vi "Email Alert (SubVI).vi"(6 "Password":string, 9 "Email":string, 10 "Phone Number":string, 11 "Carrier":enum16{"Sprint", "Verizon", "AT&T", "T-Mobile"}(ring)) -> (0 "error out":errorcluster)   [LabVIEW 2020]
uses:
  <vilib>/smtpClient/Set Message Text.vi
  <vilib>/smtpClient/LabVIEWSMTPClient.lvlib
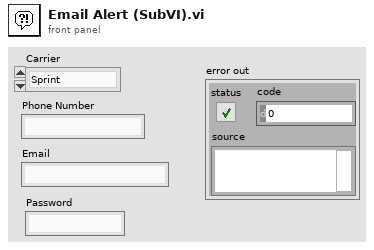
[diagram p1: front panel]
types:
  T1 = typedef "LabVIEWSMTPClient.lvlib/SmtpClientHandle.ctl" = refnum<k1>
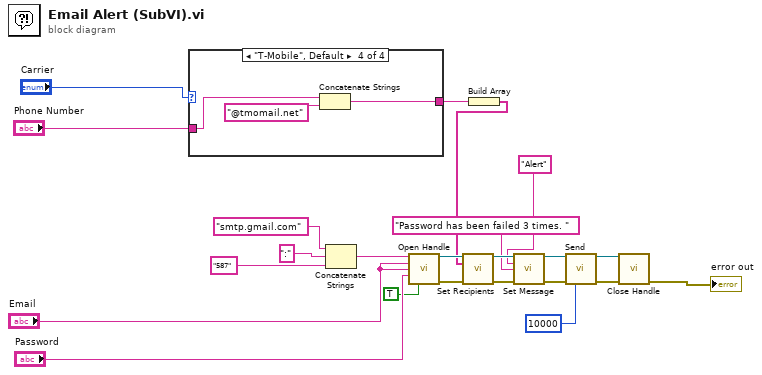
[diagram p0: block diagram]
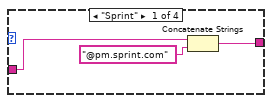
[diagram p2: hidden frame]
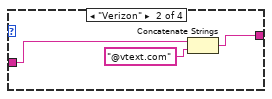
[diagram p3: hidden frame]
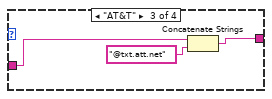
[diagram p4: hidden frame]
diagram:
  n1 = case shown="\"T-Mobile\", Default" "Carrier" {
    tunnel: "Phone Number" -> [w25 w28 w31 w35]
    tunnel: [w24 w27 w30 w33] -> w21
    frame "Sprint" {
      n2 = Concatenate Strings(w25, "@pm.sprint.com" ("string")) -> (w24:string)
    }
    frame "Verizon" {
      n3 = Concatenate Strings(w28, "@vtext.com" ("string")) -> (w27:string)
    }
    frame "AT&T" {
      n4 = Concatenate Strings(w31, "@txt.att.net" ("string")) -> (w30:string)
    }
    frame "T-Mobile", Default {
      n5 = Concatenate Strings(w35, "@tmomail.net" ("string")) -> (w33:string)
    }
  }
  n6 = Concatenate Strings("smtp.gmail.com" ("Outgoing Mail Server"), ":" ("string"), "587" ("string")) -> (w17:string)
  n7 = call <vilib>:"Open Handle.vi"("server address"=w17, "from"="Email", "username"="Email", "password"="Password", "use TLS (false)"=TRUE) -> ("handle out"=w14:T1, "error out"=w13:errorcluster)  [unwired: 9 in]
  n8 = Build Array(w21) -> (w12:string[])
  n9 = call <vilib>:"Set Recipients.vi"("handle in"=w14, "to"=w12, "error in (no error)"=w13) -> ("handle out"=w11:T1, "error out"=w10:errorcluster)  [unwired: 11 in]
  n10 = call-poly <vilib>:"Set Message.vi"("handle in"=w11, "subject"="Alert" ("Subject"), "plain text message"="Password has been failed 3 times. " ("Body"), "error in (no error)"=w10) -> ("handle out"=w7:T1, "error out"=w6:errorcluster)  [unwired: 10 in]
  n11 = call <vilib>:"Send.vi"("handle in"=w7, "error in (no error)"=w6, "timeout in ms (10000)"=10000) -> ("handle out"=w4:T1, "error out"=w3:errorcluster)  [unwired: 10 in, 1 out]
  n12 = call <vilib>:"Close Handle.vi"("handle in"=w4, "error in (no error)"=w3) -> ("error out"=→"error out":errorcluster)  [unwired: 12 in, 1 out]
